vi "Update Vehicle Out of Position.vi"(8 "error in (no error)":errorcluster, 10 "Out of pos?":bool, 11 "Simulated Wash Display Console Actor in":refnum<class "Simulated Wash Display Console Actor.lvclass">) -> (0 "error out":errorcluster, 3 "Simulated Wash Display Console Actor out":refnum<class "Simulated Wash Display Console Actor.lvclass">)   [LabVIEW 2019, in "Simulated Wash Display Console Actor.lvlib" / "Simulated Wash Display Console Actor.lvclass"]
uses:
  Simulated Wash Display Console Actor.lvclass
  Simulated Wash Display Console Actor.lvclass/Simulated Wash Display Console Actor.ctl
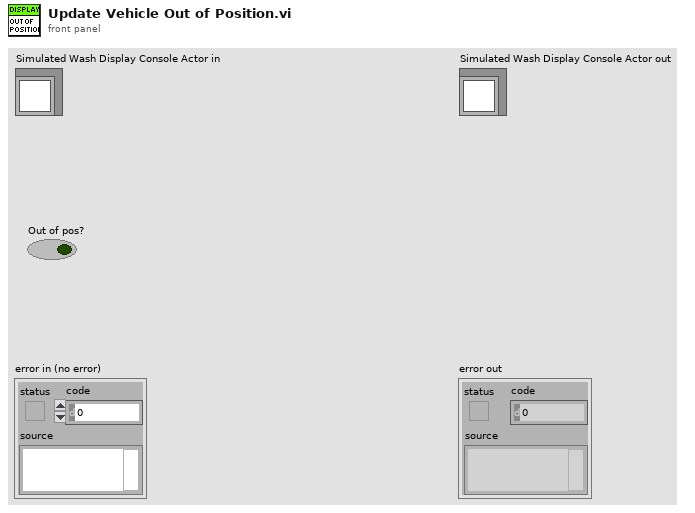
[diagram p1: front panel]
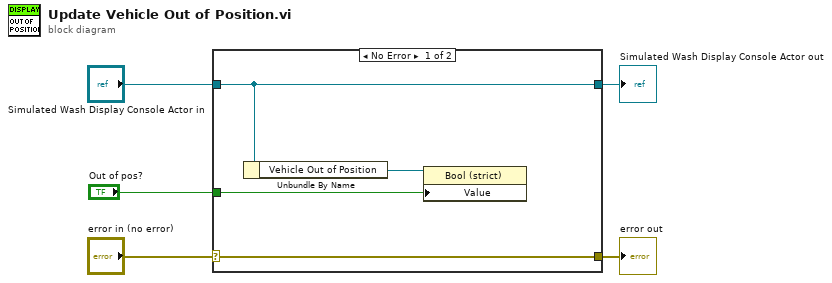
[diagram p0: block diagram]
diagram:
  n1 = case shown="No Error" "error in (no error)" {
    selector: "error in (no error)" -> [w9 w10]
    tunnel: [w9 w10] -> w4
    tunnel: [w8 w11] -> w2
    tunnel: "Simulated Wash Display Console Actor in" -> [w8 w11]
    tunnel: "Out of pos?" -> [w6 _]
    frame No Error {
      n2 = Unbundle By Name(w8) -> ("Vehicle Out of Position"=w7:refnum<vi>)
      n3 = property class="Bool (strict)"(reference=w7, "Value"=w6) -> ()  [unwired: 1 in, 2 out]
    }
    frame Error {
    }
  }
  "error out" <- w4
  "Simulated Wash Display Console Actor out" <- w2
